vi "Waveform Attribute, Set MD5.vi"(5 "MD5":string="3da10dbfb34247d8b76754de4a8a0a76", 6 "error in":errorcluster, 9 "waveform":waveform(dbl)) -> (0 "error out":errorcluster, 3 "waveform out":waveform(dbl))   [LabVIEW 2010]
doc: "This function stores an MD5 message-digest as waveform attributes. \n\nThe input message digest string is converted to four double precision floating point values and stored as four attributes (MD5[0], MD5[1], MD5[2, and MD5[3]). An MD5 empty string will write all zeroes.\n\nThe inverse of this function is \"MD5, Waveform Attribute, Get MD5.vi\""
panel:
  out "MD5[3]":dbl=nan format="%.1f"
  out "MD5[2]":dbl=nan format="%.1f"
  out "MD5[1]":dbl=nan format="%.1f"
  out "MD5[0]":dbl=nan format="%.1f"
  # "Waveform Attributes"
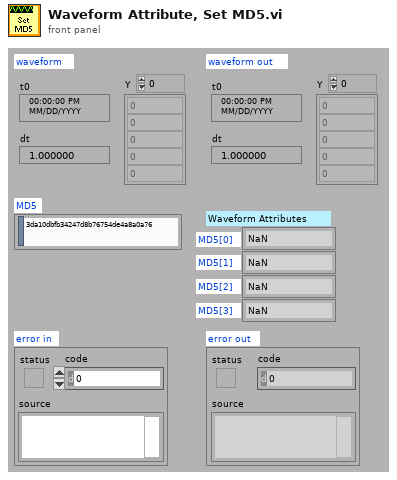
[diagram p1: front panel]
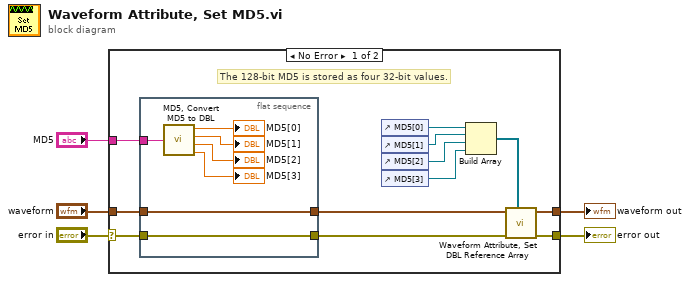
[diagram p0: block diagram]
diagram:
  n1 = case shown="No Error" "error in" {
    selector: "error in" -> [w8 w25]
    tunnel: [w16 w25] -> w5
    tunnel: [w15 _] -> w3
    tunnel: "MD5" -> [w17 _]
    tunnel: "waveform" -> [w10 _]
    frame No Error {
      # "The 128-bit MD5 is stored as four 32-bit values."
      n2 = flat-sequence {
        tunnel: w17 -> [w23]
        tunnel: w10 -> [w19]
        tunnel: [w19] -> w9
        tunnel: w8 -> [w18]
        tunnel: [w18] -> w7
        frame #0 {
          n3 = call "MD5, Convert MD5 to DBL.vi"("MD5"=w23) -> ("MD5[0]"=→"MD5[0]":dbl, "MD5[1]"=→"MD5[1]":dbl, "MD5[2]"=→"MD5[2]":dbl, "MD5[3]"=→"MD5[3]":dbl)  [unwired: 1 out]
        }
      }
      n4 = control-ref of="MD5[0]"() -> (w14:refnum<vi>)
      n5 = control-ref of="MD5[1]"() -> (w13:refnum<vi>)
      n6 = control-ref of="MD5[2]"() -> (w12:refnum<vi>)
      n7 = control-ref of="MD5[3]"() -> (w11:refnum<vi>)
      n8 = Build Array(w14, w13, w12, w11) -> (w6:refnum<vi>[])
      n9 = call "Waveform Attribute, Set DBL Reference Array.vi"("Refnum Array"=w6, "error in"=w7, "waveform"=w9) -> ("error out"=w16:errorcluster, "waveform out"=w15:waveform(dbl))  [unwired: 5 in]
    }
    frame Error {
    }
  }
  "error out" <- w5
  "waveform out" <- w3
